vi "Read Exit.vi"(8 "error in (no error)":errorcluster, 11 "PD-Data in":refnum<class "SC-Main.lvclass">) -> (0 "error out":errorcluster, 2 "Exit":refnum<notifier>, 3 "PD-Data out":refnum<class "SC-Main.lvclass">)   [LabVIEW 2013, in "SLMControl.lvlib" / "SC-Main.lvclass"]
uses:
  SC-Main.lvclass
  SC-Main.lvclass/SC-Main.ctl
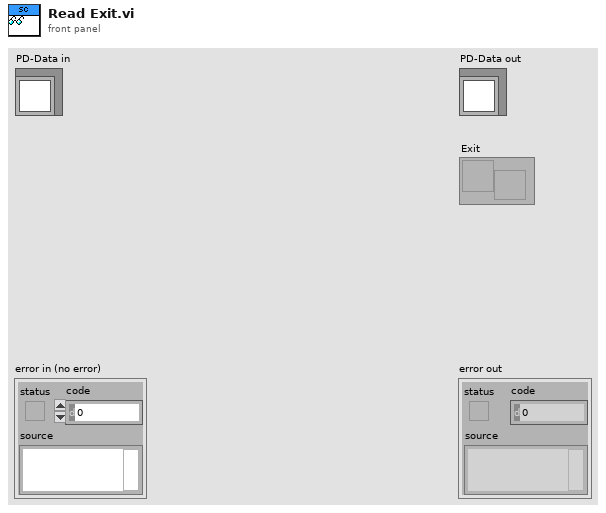
[diagram p1: front panel]
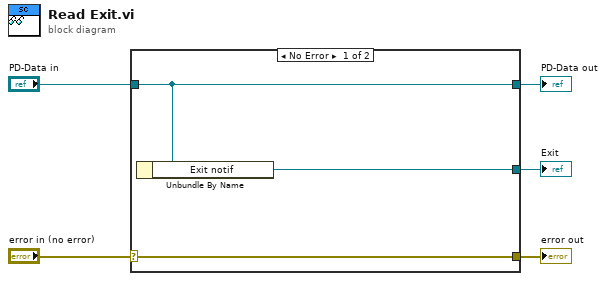
[diagram p0: block diagram]
diagram:
  n1 = case shown="No Error" "error in (no error)" {
    selector: "error in (no error)" -> [w8 w9]
    tunnel: [w8 w9] -> w4
    tunnel: [w7 w10] -> w2
    tunnel: "PD-Data in" -> [w7 w10]
    tunnel: [w6 _] -> w1
    frame No Error {
      n2 = Unbundle By Name(w7) -> ("Exit notif"=w6:refnum<notifier>)
    }
    frame Error {
    }
  }
  "error out" <- w4
  "PD-Data out" <- w2
  "Exit" <- w1
